vi "NBFM Modulation Demo (Single Tone) - SingleTone.vi"() -> ()   [LabVIEW 2013]
uses:
  <vilib>/addons/Modulation/Analog/MT Passband PLL.vi
  <vilib>/express/express analysis/Spectral/Block/exnSpectralBlock spectral measurements power poly.vi
  <vilib>/express/express analysis/Spectral/Block/exnSpectralBlock spectral measurements power DDT.vi
  <vilib>/express/express analysis/Spectral/XNode/ExpressSpectralMeasurementsBlockNode.xnode
  <vilib>/addons/Modulation/niAMT.lvlib
  <vilib>/Analysis/NI_AALPro.lvlib
panel:
  in  "Mod. Freq.":dbl=2000.0 caption="Frequency"
  out "Baseband":dynamicdata(graph)
  out "estimated carrier frequency (Hz)":dbl
  in  "WAV SR":dbl=44100.0 caption="dt"
  in  "LPF Cut-Off":dbl=10000.0 caption="Lower Cut-Off"
  in  "AWGN (dB)":dbl(slide)=30.0 caption="Standard deviation" scale=-20.0..50.0
  out "Recovered Signal":dynamicdata(graph)
  out "FM FFT":dynamicdata(graph)
  out "FM Wave":dynamicdata(graph)
  in  "Carrier Amp.":dbl=1.0 caption="Amplitude"
  in  "stop":bool
  in  "Frequency Deviation":dbl(slide)=400.0 scale=0.0..1000.0
  in  "Carrier Freq.":dbl=100000.0 caption="Frequency"
  # "Frequency Modulation"
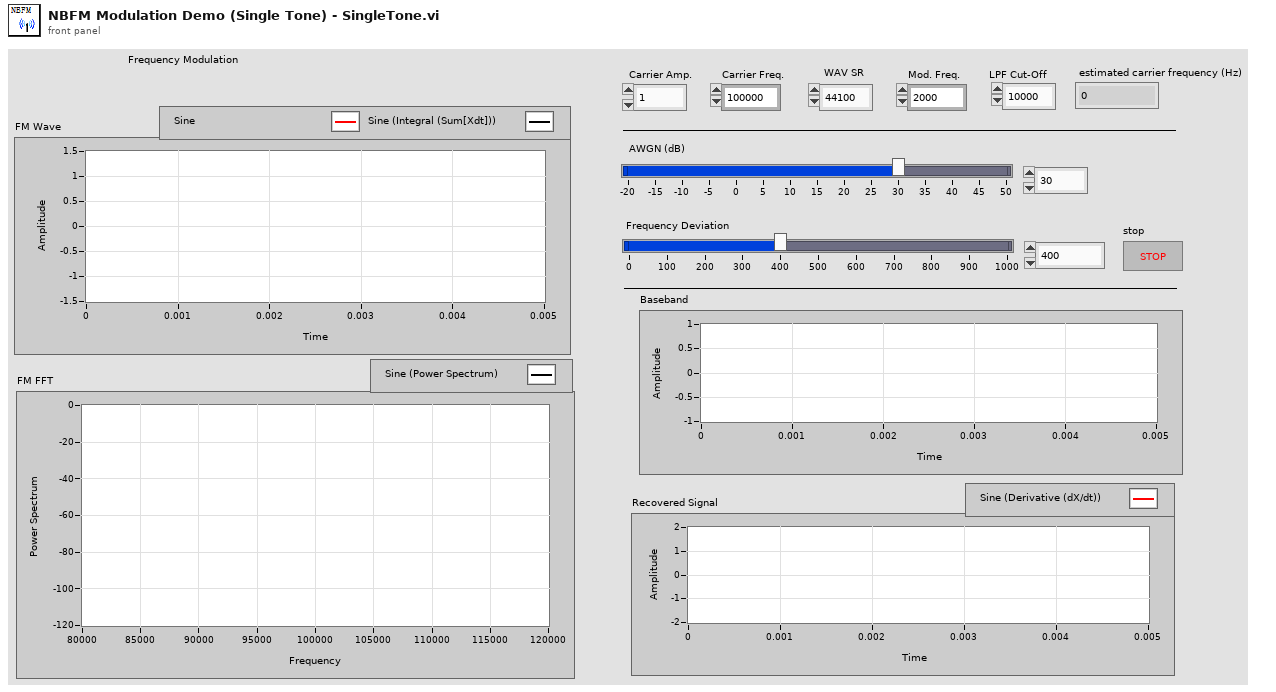
[diagram p1: front panel]
types:
  T1 = cluster{"averaging mode":u16, "weighting mode":u16, "number of averages":u32}
  T2 = cluster{"dB On (F)":bool, "unwrap phase (F)":bool, "convert to degree (F)":bool}
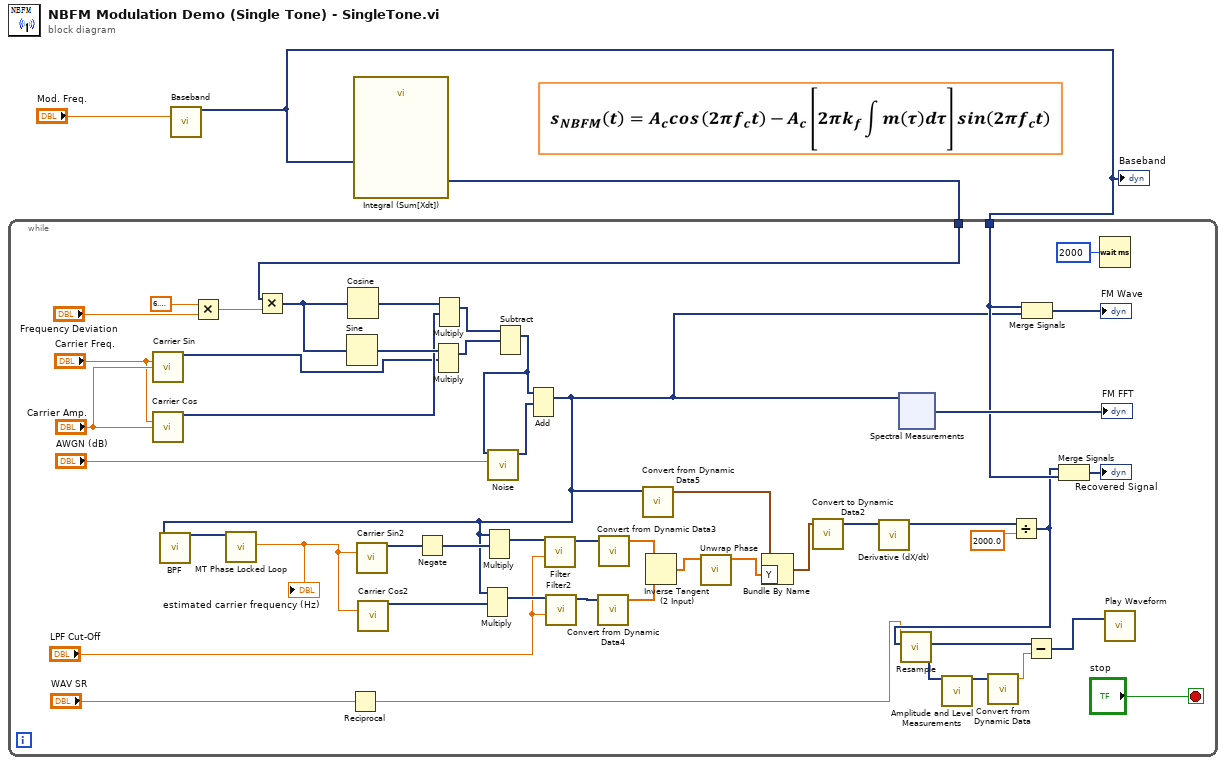
[diagram p0: block diagram]
diagram:
  n1 = call "Baseband"("Frequency"="Mod. Freq.") -> ("Sine"=w1:dynamicdata)  [unwired: 13 in, 1 out]
  "Baseband" <- w1
  n2 = call "Integral (Sum[Xdt])"("Signals"=w1) -> ("Result"=w2:dynamicdata)  [unwired: 5 in, 1 out]
  n3 = while {
    tunnel: w1 -> [w21]
    tunnel: w2 -> [w35]
    stop <- "stop" stop-if-true
    n4 = call "Carrier Sin"("Frequency"="Carrier Freq.", "Amplitude"="Carrier Amp.") -> ("Sine"=w30:dynamicdata)  [unwired: 12 in, 1 out]
    n5 = call "Carrier Cos"("Frequency"="Carrier Freq.", "Amplitude"="Carrier Amp.") -> ("Sine"=w31:dynamicdata)  [unwired: 12 in, 1 out]
    n6 = Multiply(x=6.283185307179586, y="Frequency Deviation") -> (x*y=w47:dbl)
    n7 = Multiply(x=w35, y=w47) -> (x*y=w33:dynamicdata)
    n8 = Sine(x=w33) -> (sin(x)=w32:dynamicdata)
    n9 = Cosine(x=w33) -> (cos(x)=w34:dynamicdata)
    n10 = Reciprocal(x="WAV SR") -> (1/x=w18:dbl)
    n11 = Multiply(1:w30, 2:w32) -> (0:w28:dynamicdata)  [unwired: 1 in, 1 out]
    n12 = Multiply(1:w31, 2:w34) -> (0:w29:dynamicdata)  [unwired: 1 in, 1 out]
    n13 = Subtract(1:w28, 2:w29) -> (0:w26:dynamicdata)  [unwired: 1 in, 1 out]
    n14 = call "Noise.vi"("AWGN (dB)"="AWGN (dB)", "Dynamic Data"=w26) -> ("DC with Gaussian Noise"=w27:dynamicdata)  [unwired: 9 in]
    n15 = Add(1:w27, 2:w26) -> (0:w10:dynamicdata)  [unwired: 1 in, 1 out]
    n16 = call "BPF"("Signal"=w10) -> ("Filtered Signal"=w42:dynamicdata)  [unwired: 9 in, 1 out]
    n17 = call-poly <vilib>:"MT Phase Locked Loop.vi"("passband waveform"=w42) -> ("estimated carrier frequency (Hz)"=w25:dbl)  [unwired: 10 in, 4 out]
    "estimated carrier frequency (Hz)" <- w25
    n18 = call "Carrier Sin2"("Frequency"=w25) -> ("Sine"=w41:dynamicdata)  [unwired: 13 in, 1 out]
    n19 = call "Carrier Cos2"("Frequency"=w25) -> ("Sine"=w23:dynamicdata)  [unwired: 13 in, 1 out]
    n20 = Negate(x=w41) -> (-x=w24:dynamicdata)
    n21 = Multiply(1:w23, 2:w10) -> (0:w17:dynamicdata)  [unwired: 1 in, 1 out]
    n22 = Multiply(1:w24, 2:w10) -> (0:w16:dynamicdata)  [unwired: 1 in, 1 out]
    n23 = call "Filter"("Lower Cut-Off"="LPF Cut-Off", "Signal"=w16) -> ("Filtered Signal"=w14:dynamicdata)  [unwired: 8 in, 1 out]
    n24 = call "Filter2"("Lower Cut-Off"="LPF Cut-Off", "Signal"=w17) -> ("Filtered Signal"=w13:dynamicdata)  [unwired: 8 in, 1 out]
    n25 = call "Convert from Dynamic Data4"("Dynamic Data Type"=w13) -> ("Array"=w11:dbl[])  [unwired: 3 in]
    n26 = call "Convert from Dynamic Data3"("Dynamic Data Type"=w14) -> ("Array"=w12:dbl[])  [unwired: 3 in]
    n27 = call "Convert from Dynamic Data5"("Dynamic Data Type"=w10) -> ("Waveform"=w6:waveform(dbl))  [unwired: 3 in]
    n28 = Inverse Tangent (2 Input)(1:w11, 2:w12) -> (0:w8:dbl[])
    n29 = call <vilib>:"Unwrap Phase.vi"("Phase"=w8) -> ("Unwrapped Phase"=w7:dbl[])  [unwired: 9 in, 1 out]
    n30 = Bundle By Name(cluster=w6, "Y"=w7) -> (w5:waveform(dbl))
    n31 = call "Convert to Dynamic Data2"("Waveform"=w5) -> ("Dynamic Data Type"=w9:dynamicdata)  [unwired: 3 in]
    n32 = call "Derivative (dX/dt)"("Signals"=w9) -> ("Result"=w20:dynamicdata)  [unwired: 5 in, 1 out]
    n33 = xnode "Spectral Measurements"("Signals"=w10) -> ("Power Spectrum"=→"FM FFT":dynamicdata)  [unwired: 1 in, 1 out]
    n34 = Divide(x=w20, y=2000.0) -> (x/y=w19:dynamicdata)
    n35 = call "Resample"("dt"=w18, "Signals"=w19) -> ("Resampled Signals"=w38:dynamicdata)  [unwired: 7 in, 2 out]
    n36 = call "Amplitude and Level Measurements"("Signals"=w38) -> ("Mean (DC)"=w39:dynamicdata)  [unwired: 13 in, 1 out]
    n37 = call "Convert from Dynamic Data"("Dynamic Data Type"=w39) -> ("Scalar"=w37:dbl)  [unwired: 3 in]
    n38 = Merge Signals(w21, w10) -> (→"FM Wave":dynamicdata)
    n39 = Subtract(x=w38, y=w37) -> (x-y=w36:dynamicdata)
    n40 = Merge Signals(w19, w21) -> (→"Recovered Signal":dynamicdata)
    n41 = Wait (ms)(milliseconds to wait=u32 2000) -> ()  [unwired: 1 out]
    n42 = call "Play Waveform"("Data"=w36) -> ()  [unwired: 18 in, 1 out]
  }
